vi "9870 Interface DMA (FPGA).vi"() -> ()   [LabVIEW 2022 SP3]
uses:
  FPGA Function.ctl
  <vilib>/rvi/Emulation/niFpgaGetClockAttributes.vi
  <vilib>/rvi/Emulation/niFpgaSctlEmulationGetInTimedLoop.vi
  <vilib>/rvi/Emulation/niFpgaEmulationReportErrorSimple.vi
  <vilib>/rvi/eio/common/nirviEmuTemplateMethod_errors.vi
  <vilib>/rvi/interface/RandomDataEmulation/niFpgaRandomDataHandleErrors.vi
  <vilib>/rvi/Emulation/niFpgaCriticalErrorInLSC.vi
  <vilib>/eio/EIOMethodNode/EIOMethodNode.xnode
  <vilib>/rvi/DataTransferAndStorage/Container/XNode/niFpgaContainer.xnode
  <vilib>/rvi/interface/RandomDataEmulation/nirviRandomDataFpgaReadWriteTemplate.vi
panel:
  out "EOS?":bool
  in  "EOS Enabled":bool
  in  "EOS":u8
  in  "Byte Timeout":i32=10
  in  "error in":errorcluster
  in  "Op Control":T1
  out "Timed Out":bool
  out "error out":errorcluster
  in  "Number of Bytes":i32=1
  # "WRITE"
  # "READ"
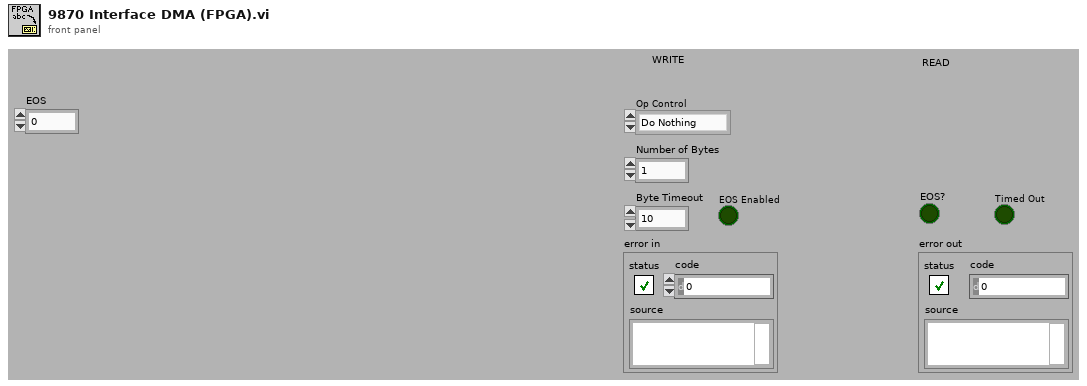
[diagram p1: front panel]
types:
  T1 = typedef "FPGA Function.ctl" = enum16{"Do Nothing", "Write", "Read"}
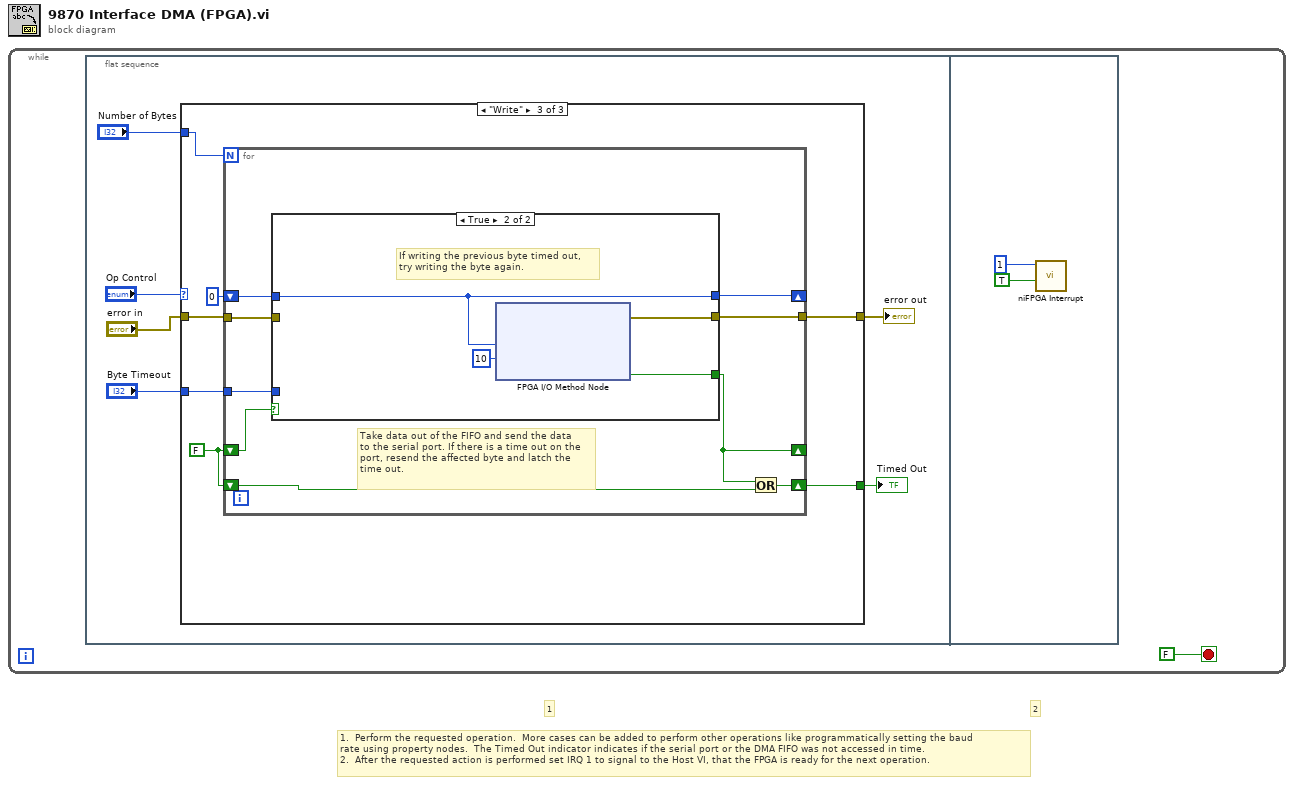
[diagram p0: block diagram]
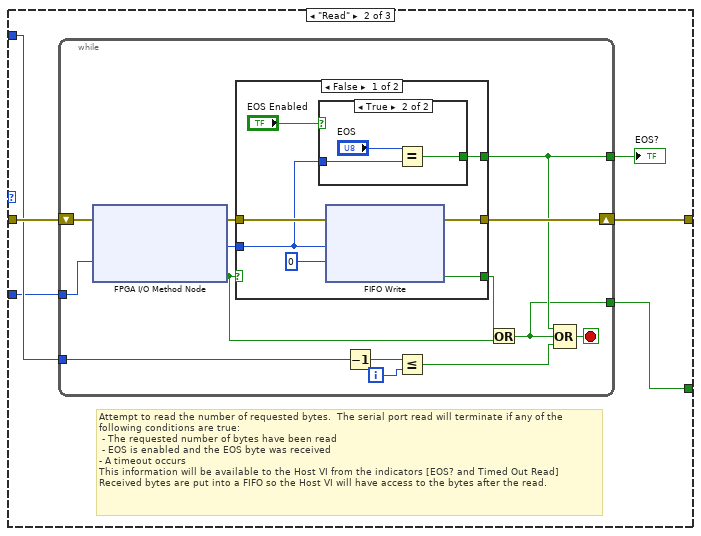
[diagram p3: hidden frame]
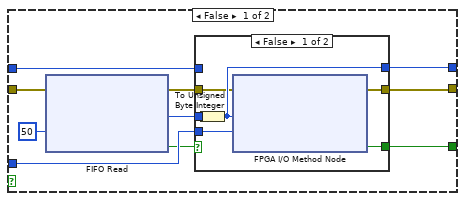
[diagram p6: hidden frame]
diagram:
  # "2"
  # "1"
  # "1.  Perform the requested operation.  More cases can be added to perform other operations like programmatically setting the baud \nrate using property nodes.  The Timed Out indicator indicates if the serial port or the DMA FIFO was not accessed in time.\n2.  After the requested action is performed set IRQ 1 to signal to the Host VI, that the FPGA is ready for the next operation."
  n1 = while {
    stop <- FALSE stop-if-true
    n2 = flat-sequence {
      frame #0 {
        n3 = case shown="\"Write\"" "Op Control" {
          tunnel: "Number of Bytes" -> [_ w12 w48]
          tunnel: [w8 w14 w47] -> w5
          tunnel: "error in" -> [w8 w13 w45]
          tunnel: "Byte Timeout" -> [_ w10 w44]
          tunnel: [_ w11 w42] -> w2
          frame "Do Nothing", Default {
          }
          frame "Read" {
            # "Attempt to read the number of requested bytes.  The serial port read will terminate if any of the \nfollowing conditions are true:\n - The requested number of bytes have been read\n - EOS is enabled and the EOS byte was received\n- A timeout occurs\nThis information will be available to the Host VI from the indicators [EOS? and Timed Out Read]\nReceived bytes are put into a FIFO so the Host VI will have access to the bytes after the read."
            n4 = while {
              tunnel: w12 -> [w23]
              shift-right: [w28] -> w14
              shift-left: w13 -> [w26]
              tunnel: [w16] -> w11
              tunnel: w10 -> [w19]
              tunnel: [w17] -> w9
              i -> [w22]
              stop <- w21 stop-if-true
              n5 = xnode "FPGA I/O Method Node"("error in"=w26, "Timeout (ms)"=w19) -> ("error out"=w27:errorcluster, "Data"=w25:u8, "Timed Out"=w18:bool)  [unwired: 1 in, 1 out]
              n6 = case shown="False" w18 {
                selector: w18 -> [_ w40]
                tunnel: [w35 w40] -> w20
                tunnel: w25 -> [w30 _]
                tunnel: [w33 w41] -> w28
                tunnel: w27 -> [w32 w41]
                tunnel: [w29 _] -> w17
                frame False {
                  n7 = case shown="True" "EOS Enabled" {
                    selector: "EOS Enabled" -> [w36 _]
                    tunnel: w30 -> [_ w39]
                    tunnel: [w36 w37] -> w29
                    frame False {
                    }
                    frame True {
                      n8 = Equal?(x="EOS", y=w39) -> (x = y?=w37:bool)
                    }
                  }
                  n9 = xnode ("FIFO Write")("Element"=w30, "Timeout"=0, "error in (no error)"=w32) -> ("Timed Out?"=w35:bool, "error out"=w33:errorcluster)  [unwired: 1 in, 1 out]
                }
                frame True {
                }
              }
              n10 = Decrement(x=w23) -> (x-1=w24:i32)
              n11 = Less Or Equal?(x=w24, y=w22) -> (x <= y?=w15:bool)
              n12 = Or(x=w20, y=w18) -> (x .or. y?=w16:bool)
              n13 = Compound Arithmetic op=OR(w17, w16, w15) -> (w21:bool)
            }
            "EOS?" <- w9
          }
          frame "Write" {
            w43 = FALSE ("Timed Out")
            n14 = for {
              N: w48 -> [_]
              tunnel: [w57] -> w47
              shift-right: [w55] -> _
              shift-left: u8 0 ("Byte to write") -> [w56]
              tunnel: w45 -> [w52]
              shift-right: [w50] -> _
              shift-left: w43 -> [w54]
              tunnel: w44 -> [w53]
              shift-right: [w51] -> w42
              shift-left: w43 -> [w49]
              # "Take data out of the FIFO and send the data\nto the serial port. If there is a time out on the\nport, resend the affected byte and latch the\ntime out."
              n15 = case shown="True" w54 {
                tunnel: [w67 w79] -> w57
                tunnel: [w66 w78] -> w50
                tunnel: w56 -> [w58 w76]
                tunnel: [w65 w76] -> w55
                tunnel: w53 -> [w64 _]
                tunnel: w52 -> [w62 _]
                frame False {
                  n16 = xnode ("FIFO Read")("Timeout"=50, "error in (no error)"=w62) -> ("Element"=w60:i16, "Timed Out?"=w59:bool, "error out"=w61:errorcluster)  [unwired: 1 in, 1 out]
                  n17 = case shown="False" w59 {
                    tunnel: [w73 w75] -> w67
                    tunnel: [w72 _] -> w66
                    tunnel: [w71 w74] -> w65
                    tunnel: w64 -> [w70 _]
                    tunnel: w61 -> [w69 w75]
                    tunnel: w60 -> [w68 _]
                    tunnel: w58 -> [_ w74]
                    frame False {
                      n18 = To Unsigned Byte Integer(number=w68) -> (unsigned 8bit integer=w71:u8)
                      n19 = xnode "FPGA I/O Method Node"("error in"=w69, "Data"=w71, "Timeout (ms)"=w70) -> ("error out"=w73:errorcluster, "Timed Out"=w72:bool)  [unwired: 1 in, 1 out]
                    }
                    frame True {
                    }
                  }
                }
                frame True {
                  # "If writing the previous byte timed out,\ntry writing the byte again."
                  n20 = xnode "FPGA I/O Method Node"("Data"=w76, "Timeout (ms)"=10) -> ("error out"=w79:errorcluster, "Timed Out"=w78:bool)  [unwired: 2 in, 1 out]
                }
              }
              n21 = Or(x=w50, y=w49) -> (x .or. y?=w51:bool)
            }
          }
        }
        "error out" <- w5
        "Timed Out" <- w2
      }
      frame #1 {
        n22 = call <vilib>:"niFPGA Interrupt.vi"("Wait Until Cleared (F)"=TRUE ("Wait Until Cleared"), "IRQ Number (0)"=u8 1 ("IRQ Number")) -> ()  [unwired: 1 in]
      }
    }
  }
